vi "Test_WriteValue_InvalidPath_Error.vi"(8 "error in (no error)":errorcluster, 11 "TestCase in":refnum<class "TestPersistToDiskTransport.lvclass">) -> (0 "error out":errorcluster, 3 "TestCase out":refnum<class "TestPersistToDiskTransport.lvclass">)   [LabVIEW 2017, in "TestPersistToDiskTransport.lvclass"]
uses:
  TestPersistToDiskTransport.lvclass
  Source/Concrete/PersistToDiskTransport/PersistToDiskTransport.lvclass/PersistToDiskTransport.ctl
  <vilib>/Utility/error.llb/Clear Errors.vi
  Source/Concrete/PersistToDiskTransport/PersistToDiskTransport.lvclass
  C:/Git/composed-transport/Source/ITransport/ITransport.lvclass
  Source/ITransport/ITransport.lvclass
panel:
  out "Return Error":errorcluster
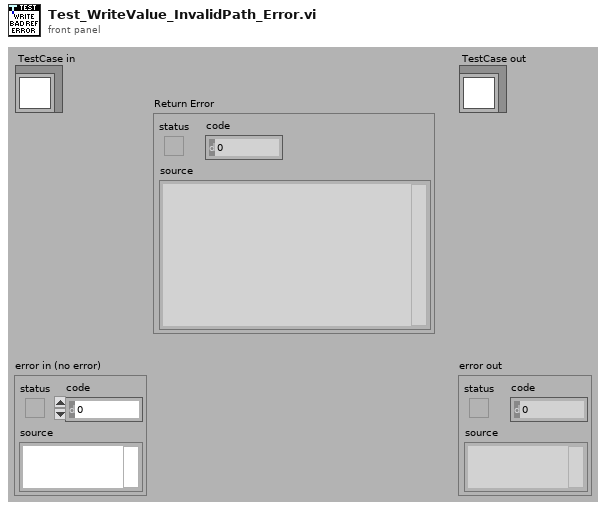
[diagram p1: front panel]
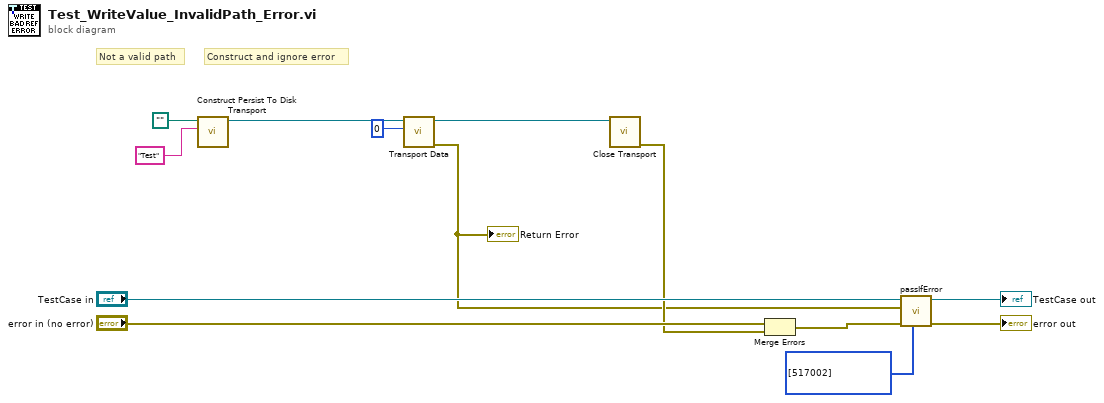
[diagram p0: block diagram]
diagram:
  # "Construct and ignore error"
  # "Not a valid path"
  n1 = call "Construct Persist To Disk Transport.vi"("Datum Name"="Test" ("Key Name"), "Folder Path"=path "") -> ("PersistToDiskTransport"=w9:refnum<class "PersistToDiskTransport.lvclass">)  [unwired: 8 in, 1 out]
  n2 = call "Transport Data.vi"("Value"=0, "ITransport in"=w9) -> ("error out"=w3:errorcluster, "ITransport out"=w4:refnum<class "PersistToDiskTransport.lvclass">)  [unwired: 8 in]
  "Return Error" <- w3
  n3 = call-dynamic "Close Transport.vi"("ITransport in"=w4) -> ("error out"=w7:errorcluster)  [unwired: 10 in]
  n4 = Merge Errors("error in (no error)", w7) -> (w10:errorcluster)
  n5 = call-dynamic "passIfError.vi"("passing error codes (default = any error code)"=i32[] [517002], "error in (no error)"=w10, "error"=w3, "TestCase in"="TestCase in") -> ("error out"=→"error out":errorcluster, "TestCase out"=→"TestCase out":refnum<class "TestPersistToDiskTransport.lvclass">)  [unwired: 6 in]
